vi "Create.vi"(8 "error in (no error)":errorcluster, 11 "baseURL":string) -> (0 "error out":errorcluster, 3 "REST_Client out":refnum<class "REST_Client.lvclass">)   [LabVIEW 2020, in "REST_Client.lvclass"]
uses:
  REST_Client.lvclass
  <vilib>/httpClient/LabVIEWHTTPClient.lvlib
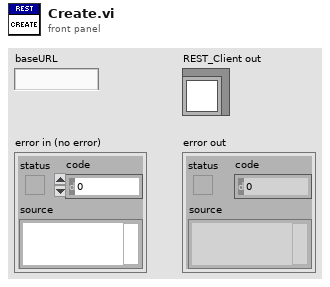
[diagram p1: front panel]
types:
  T1 = typedef "LabVIEWHTTPClient.lvlib/ClientHandle.ctl" = refnum<k1>
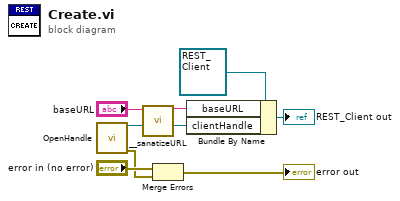
[diagram p0: block diagram]
diagram:
  n1 = call <vilib>:"OpenHandle.vi"() -> ("client handle out"=w7:T1, "error out"=w5:errorcluster)  [unwired: 14 in]
  n2 = call "__sanatizeURL.vi"("url in"="baseURL") -> ("url out"=w1:string)  [unwired: 10 in]
  n3 = Merge Errors("error in (no error)", w5) -> (→"error out":errorcluster)
  n4 = Bundle By Name(cluster=refnum<class "REST_Client.lvclass"> refnum ("REST_Client.lvclass"), "baseURL"=w1, "clientHandle"=w7) -> (→"REST_Client out":refnum<class "REST_Client.lvclass">)
